vi "rvc draw cylinder between two points.vi"(6 "Color":T1={"Red"=1.0, "Green"=0.0, "Blue"=1.0, "Alpha"=1.0}, 7 "Name":string="asdf", 9 "radius":dbl, 10 "Point B":dbl[](array[numeric]), 11 "Point A":dbl[](array[numeric])) -> (3 "Rotated Scene Object":refnum<vi>)   [LabVIEW 2013]
uses:
  <vilib>/Analysis/baseanly.llb/Unit Vector (DBL).vi
  <vilib>/Analysis/baseanly.llb/Real Dot Product.vi
  <vilib>/picture/3D Picture Control/Object/Create Object (name).vi
  <vilib>/picture/3D Picture Control/Object/Create Object (drawable).vi
  <vilib>/picture/3D Picture Control/NI_3D Picture Control.lvlib
  <vilib>/Analysis/NI_AALBase.lvlib
  <vilib>/Analysis/NI_AALPro.lvlib
panel:
  out "error out":errorcluster
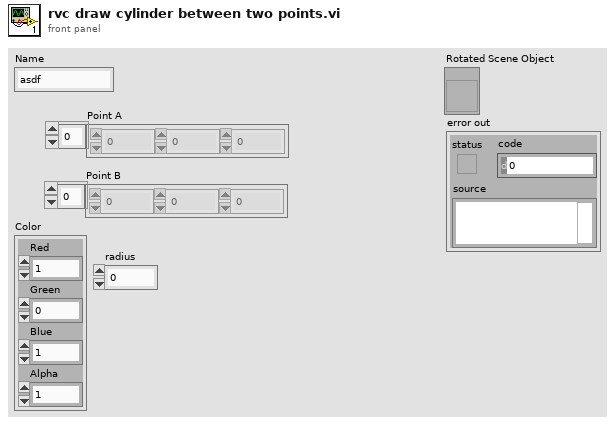
[diagram p1: front panel]
types:
  T1 = cluster{"Red":sgl, "Green":sgl, "Blue":sgl, "Alpha":sgl}
  T2 = cluster{"Cross Product[0]":dbl, "Cross Product[1]":dbl, "Cross Product[2]":dbl}
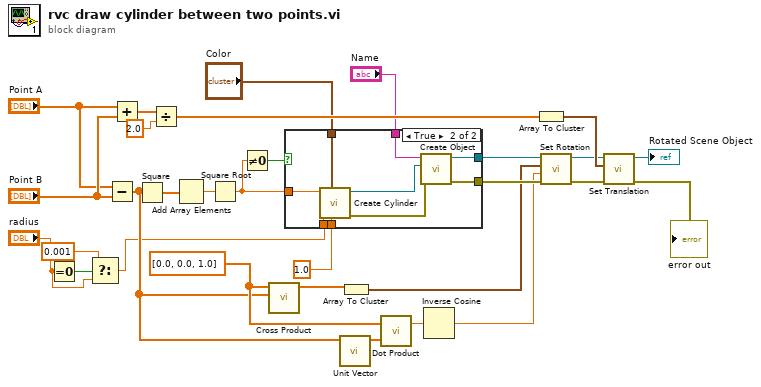
[diagram p0: block diagram]
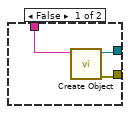
[diagram p2: hidden frame]
diagram:
  w12 = dbl[] [0.0, 0.0, 1.0] ("vector")
  n1 = Equal To 0?(x="radius") -> (x = 0?=w8:bool)
  n2 = Select(t=0.001, s=w8, f="radius") -> (s? t:f=w6:dbl)
  n3 = Subtract(x="Point A", y="Point B") -> (x-y=w11:dbl[])
  n4 = Add(x="Point A", y="Point B") -> (x+y=w17:dbl[])
  n5 = Square(x=w11) -> (x^2=w25:dbl[])
  n6 = Divide(x=w17, y=2.0) -> (x/y=w27:dbl[])
  n7 = Add Array Elements(numeric array=w25) -> (sum=w30:dbl)
  n8 = Square Root(x=w30) -> (sqrt(x)=w3:dbl)
  n9 = Not Equal To 0?(x=w3) -> (x != 0?=w2:bool)
  n10 = call <vilib>:"Cross Product.vi"("B Vector"=w11, "A Vector"=w12) -> ("Cross Product"=w10:dbl[])  [unwired: 8 in, 1 out]
  n11 = case shown="True" w2 {
    tunnel: sgl 1.0 ("Detail") -> [_ w41]
    tunnel: "Name" -> [w31 w40]
    tunnel: [w33 w39] -> w21
    tunnel: [w32 w37] -> w18
    tunnel: w6 -> [_ w36]
    tunnel: w3 -> [_ w35]
    tunnel: "Color" -> [_ w34]
    frame False {
      n12 = call-poly <vilib>:"Create Object.vi"("Name"=w31) -> ("error out"=w33:errorcluster, "Scene:New Object"=w32:refnum<vi>)  [unwired: 9 in]
    }
    frame True {
      n13 = call <vilib>:"Create Cylinder.vi"("Detail"=w41, "Color"=w34, "Radius"=w36, "Height"=w35) -> ("error out"=w38:errorcluster, "New Cylinder Refnum"=w42:refnum<vi>)  [unwired: 1 in, 5 out]
      n14 = call-poly <vilib>:"Create Object.vi"("error in (no error)"=w38, "Geometry"=w42, "Name"=w40) -> ("error out"=w39:errorcluster, "Scene:New Object"=w37:refnum<vi>)  [unwired: 7 in]
    }
  }
  n15 = call-poly <vilib>:"Unit Vector.vi"("Input Vector"=w11) -> ("Unit Vector"=w15:dbl[])  [unwired: 8 in, 2 out]
  n16 = Array To Cluster(array=w10) -> (cluster=w9:T2)
  n17 = call-poly <vilib>:"Dot Product.vi"("Y Vector"=w15, "X Vector"=w12) -> ("X * Y"=w14:dbl)  [unwired: 1 out]
  n18 = Inverse Cosine(1:w14) -> (0:w13:dbl)
  n19 = Array To Cluster(array=w27) -> (cluster=w29:cluster{"[0]":dbl, "[1]":dbl, "[2]":dbl})
  n20 = call <vilib>:"Set Rotation.vi"("error in (no error)"=w21, "Angle"=w13, "Axis"=w9, "Scene Object"=w18) -> ("error out"=w16:errorcluster, "Rotated Scene Object"=w19:refnum<vi>)  [unwired: 6 in]
  n21 = call <vilib>:"Set Translation.vi"("error in (no error)"=w16, "Translation"=w29, "Scene Object"=w19) -> ("error out"=→"error out":errorcluster, "Translated Object"=→"Rotated Scene Object":refnum<vi>)  [unwired: 7 in]
